vi "Thermal Cam Standalone.vi"() -> ()   [LabVIEW 2025]
uses:
  CTI/Identity.ctl
  Colormaps/LV Colormap Names.ctl
  CTI/GPIO Pull.ctl
  45a22dfa-6e5d-42d3-9540-e99b2dd074d1.vi
  1e6ec9c9-fb05-4fd0-b05f-9caec19ae962.vi
  8524c294-126d-4a78-a4f4-5e8209367d85.vi
  7e432e81-cfec-40ee-91ac-c41f46aea1a5.vi
  81a0c2b0-cfce-4e0a-bc55-b9605872672a.vi
  <vilib>/gmath/interp.llb/Interpolate 2D (2d X,Y).vi
  CTI/Session/Session.lvclass
  <vilib>/gmath/NI_Gmath.lvlib
  <vilib>/ptbypt/NI_PtbyPt.lvlib
  CTI/VisaComms/VisaComms.lvclass
  CTI/CTI.lvlib
panel:
  in  "Interpolate":bool=TRUE
  in  "Max hold":bool
  in  "Temperature\nCompression":dbl=3.0
  in  "Auto Z Scale":bool=TRUE
  out "Average Max":dbl=82.15301832388433 format="%.1f"
  out "Current Max":dbl=82.15301832388433 format="%.1f"
  in  "Exponentional\nAveraging Alpha":dbl=0.4 min=0.0 max=1.0 step=0.05 format="%#_13g"
  in  "Temperature\nDispalyRange":dbl=12.0
  in  "Smoothing \nMethod":i32(ring)=3 items=["nearest", "bilinear", "bicubic", "bicubic spline"]
  in  "Colormap Name":T1=enum."turbo"
  in  "Stop":bool
  out "Unprocessed Pixels":dbl[][](graph)
  out "Interpolated Frame":dbl[][](graph)
  out "Processing Performance":dbl(graph)=0.0211100999986229
  out "Identity":T2
  out "On-board\nTempSensor":dbl
  out "Frame Count":i32
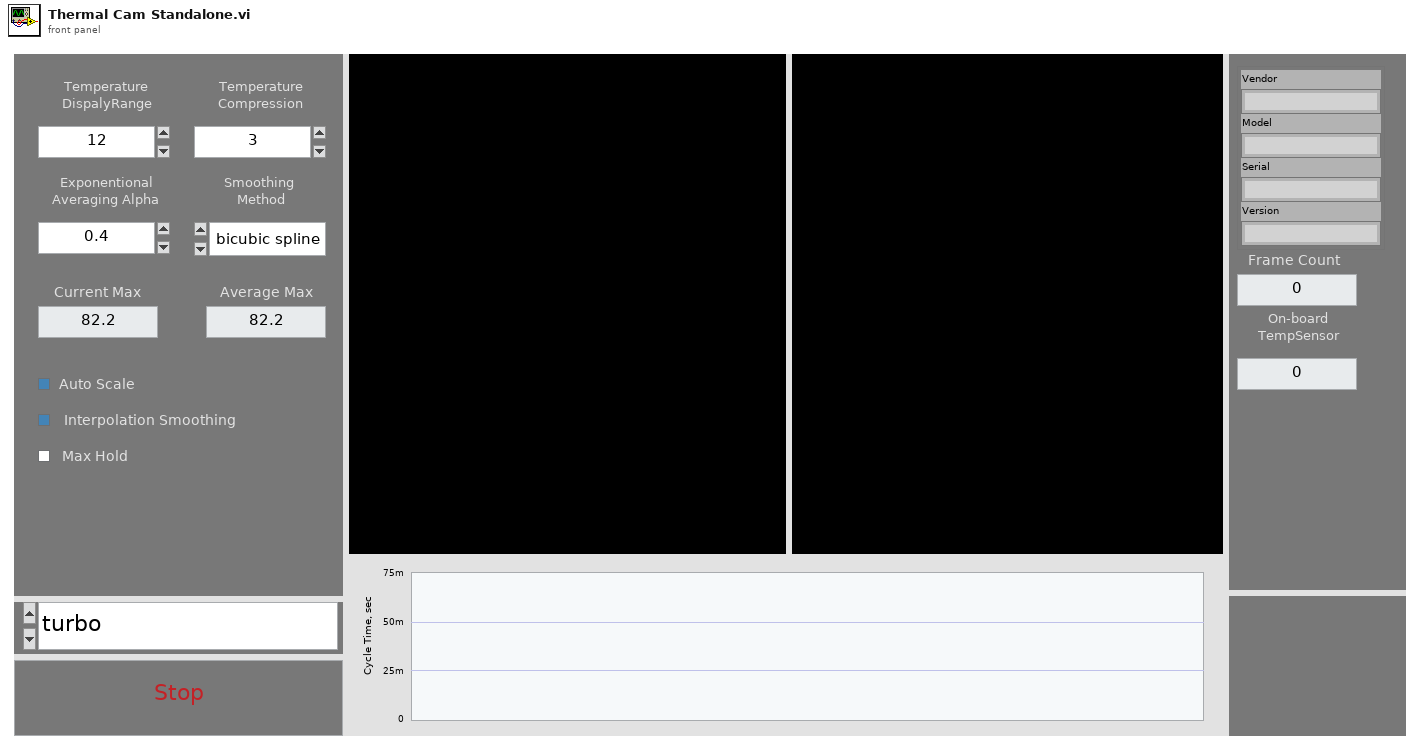
[diagram p1: front panel]
types:
  T1 = typedef "LV Colormap Names.ctl" = enum16{"Accent", "Accent_r", "Blues", "Blues_r", "BrBG", "BrBG_r", "BuGn", "BuGn_r", "BuPu", "BuPu_r", "CMRmap", "CMRmap_r", "Dark2", "Dark2_r", "GnBu", "GnBu_r", "Grays", "Grays_r", "Greens", "Greens_r", "Greys", "Greys_r", "OrRd", "OrRd_r", "Oranges", "Oranges_r", "PRGn", "PRGn_r", "Paired", "Paired_r", "Pastel1", "Pastel1_r", "Pastel2", "Pastel2_r", "PiYG", "PiYG_r", "PuBu", "PuBuGn", "PuBuGn_r", "PuBu_r", "PuOr", "PuOr_r", "PuRd", "PuRd_r", "Purples", "Purples_r", "RdBu", "RdBu_r", "RdGy", "RdGy_r", "RdPu", "RdPu_r", "RdYlBu", "RdYlBu_r", "RdYlGn", "RdYlGn_r", "Reds", "Reds_r", "Set1", "Set1_r", "Set2", "Set2_r", "Set3", "Set3_r", "Spectral", "Spectral_r", "Wistia", "Wistia_r", "YlGn", "YlGnBu", "YlGnBu_r", "YlGn_r", "YlOrBr", "YlOrBr_r", "YlOrRd", "YlOrRd_r", "afmhot", "afmhot_r", "autumn", "autumn_r", "berlin", "berlin_r", "binary", "binary_r", "bone", "bone_r", "brg", "brg_r", "bwr", "bwr_r", "cividis", "cividis_r", "cool", "cool_r", "coolwarm", "coolwarm_r", "copper", "copper_r", "cubehelix", "cubehelix_r", "flag", "flag_r", "gist_earth", "gist_earth_r", "gist_gray", "gist_gray_r", "gist_grey", "gist_grey_r", "gist_heat", "gist_heat_r", "gist_ncar", "gist_ncar_r", "gist_rainbow", "gist_rainbow_r", "gist_stern", "gist_stern_r", "gist_yarg", "gist_yarg_r", "gist_yerg", "gist_yerg_r", "gnuplot", "gnuplot2", "gnuplot2_r", "gnuplot_r", "gray", "gray_r", "grey", "grey_r", "hot", "hot_r", "hsv", "hsv_r", "inferno", "inferno_r", "jet", "jet_r", "magma", "magma_r", "managua", "managua_r", "nipy_spectral", "nipy_spectral_r", "ocean", "ocean_r", "pink", "pink_r", "plasma", "plasma_r", "prism", "prism_r", "rainbow", "rainbow_r", "seismic", "seismic_r", "spring", "spring_r", "summer", "summer_r", "tab10", "tab10_r", "tab20", "tab20_r", "tab20b", "tab20b_r", "tab20c", "tab20c_r", "terrain", "terrain_r", "turbo", "turbo_r", "twilight", "twilight_r", "twilight_shifted", "twilight_shifted_r", "vanimo", "vanimo_r", "viridis", "viridis_r", "winter", "winter_r"}
  T2 = typedef "CTI.lvlib/Identity.ctl" = cluster{"Vendor":string, "Model":string, "Serial":string, "Version":string}
  T3 = typedef "CTI.lvlib/GPIO Pull.ctl" = enum16{"None", "Up", "Down", "Both"}
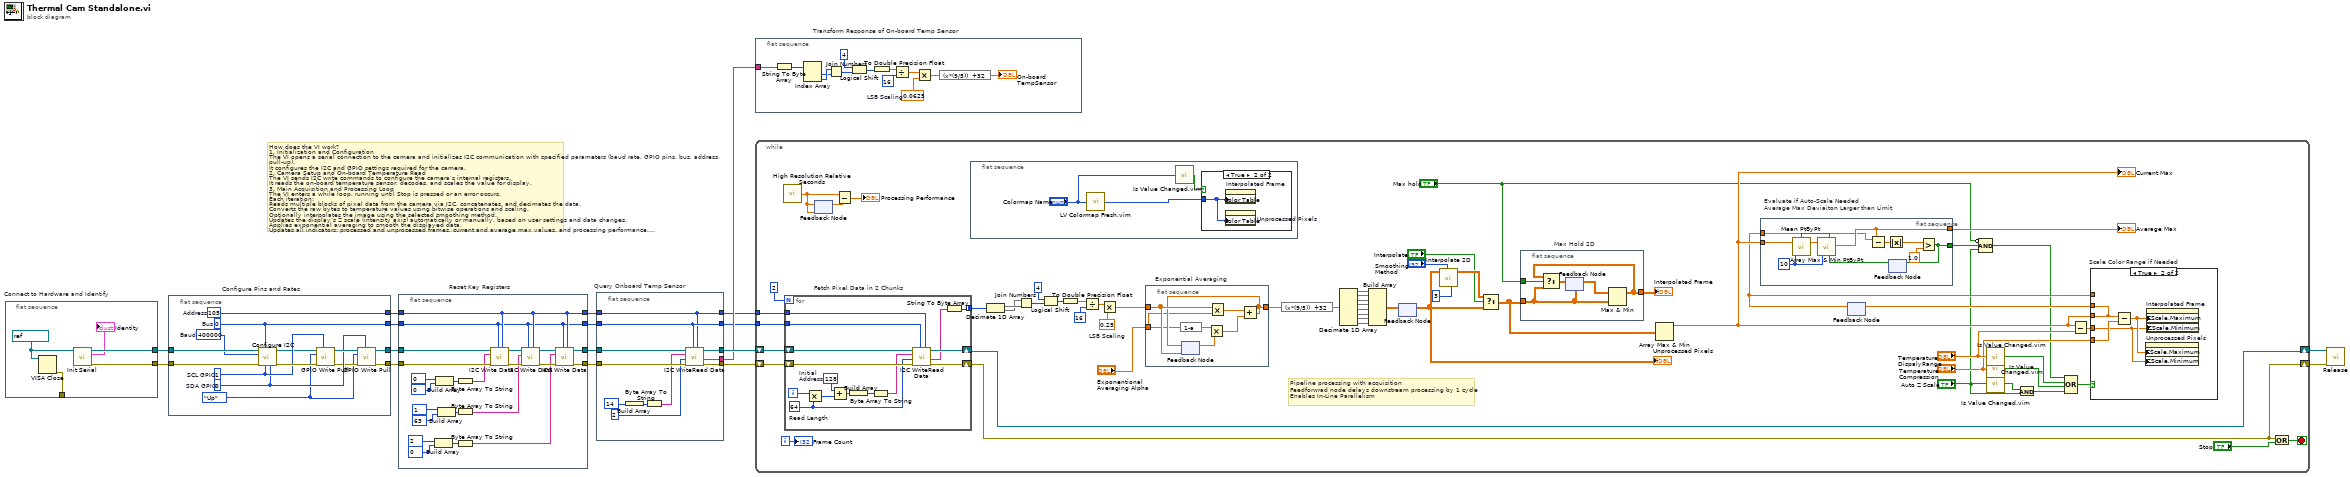
[diagram p0: block diagram]
diagram:
  # "How does the VI work?\n1. Initialization and Configuration\nThe VI opens a serial connection to the camera and initializes I2C communication with specified parameters (baud rate, GPIO pins, bus, address, pull-up).\nIt configures the I2C and GPIO settings required for the camera.\n2. Camera Setup and On-board Temperature Read\nThe VI sends I2C write commands to configure the camera’s internal registers.\nIt reads the on-board temperature sensor, decodes, and scales the value for display.\n3. Main Acquisition and Processing Loop\nThe VI enters a while loop, running until Stop is pressed or an error occurs.\nEach iteration:\nReads multiple blocks of pixel data from the camera via I2C, concatenates, and decimates the data.\nConverts the raw bytes to temperature values using bitwise operations and scaling.\nOptionally interpolates the image using the selected smoothing method.\nUpdates the display’s Z scale (intensity axis) automatically or manually, based on user settings and data changes.\nApplies exponential averaging to smooth the displayed data.\nUpdates all indicators: processed and unprocessed frames, current and average max values, and processing performance.\n4. Visualization\nThe VI updates the color map of the intensity graph if the user changes the colormap.\nIt provides options for interpolation, auto-scaling, and maximum hold to enhance visualization.\n5. Cleanup\nAfter the loop, the VI releases the camera session and cleans up resources."
  n1 = flat-sequence "Connect to Hardware and Identify" {
    tunnel: [w22] -> w17
    tunnel: [w21] -> w16
    tunnel: [w18] -> _
    frame #0 {
      w19 = refnum<visa-resource-name> "COM9" ("VISA resource name in")
      n2 = VISA Close(VISA resource name=w19) -> (error out=w18:errorcluster)  [unwired: 1 in]
      n3 = call "Init Serial.vi"("VISA resource name in"=w19) -> ("error out"=w21:errorcluster, "Identity"=→"Identity":T2, "Session"=w22:refnum<class "Session.lvclass">)  [unwired: 8 in]
    }
  }
  n4 = flat-sequence "Configure Pins and Rates" {
    tunnel: w17 -> [w36]
    tunnel: w16 -> [w35]
    tunnel: [w28] -> w15
    tunnel: [w27] -> w14
    tunnel: [w26] -> w9
    tunnel: [w25] -> w8
    frame #0 {
      w23 = GPIO_Pull."Up" ("GPIO Pull")
      w25 = u8 105  # Address
      w26 = u8 0  # Bus
      w31 = 1  # SCL GPIO
      w30 = 0  # SDA GPIO
      w34 = u32 400000  # Baud
      n5 = call "Configure I2C.vi"("SDA GPIO"=w30, "SCL GPIO"=w31, "I2C #"=w26, "error in (no error)"=w35, "Baud"=w34, "Session in"=w36) -> ("error out"=w33:errorcluster, "Session out"=w24:refnum<class "Session.lvclass">)  [unwired: 4 in]
      n6 = call "GPIO Write Pull.vi"("GPIO #"=w31, "error in (no error)"=w33, "GPIO Pull"=w23, "Session in"=w24) -> ("error out"=w29:errorcluster, "Session out"=w32:refnum<class "Session.lvclass">)  [unwired: 6 in]
      n7 = call "GPIO Write Pull.vi"("GPIO #"=w30, "error in (no error)"=w29, "GPIO Pull"=w23, "Session in"=w32) -> ("error out"=w28:errorcluster, "Session out"=w27:refnum<class "Session.lvclass">)  [unwired: 6 in]
    }
  }
  n8 = flat-sequence "Reset Key Registers" {
    tunnel: w15 -> [w58]
    tunnel: w14 -> [w57]
    tunnel: [w45] -> w13
    tunnel: [w39] -> w11
    tunnel: w9 -> [w37]
    tunnel: w8 -> [w38]
    tunnel: [w38] -> w6
    tunnel: [w37] -> w5
    frame #0 {
      n9 = Build Array(u8 2 ("Address"), u8 0 ("Address")) -> (w41:u8[])
      n10 = Build Array(u8 0 ("Address"), u8 0 ("Address")) -> (w53:u8[])
      n11 = Build Array(u8 1 ("Address"), u8 63 ("Address")) -> (w49:u8[])
      n12 = Byte Array To String(unsigned byte array=w53) -> (string=w56:string)
      n13 = Byte Array To String(unsigned byte array=w49) -> (string=w46:string)
      n14 = Byte Array To String(unsigned byte array=w41) -> (string=w40:string)
      n15 = call "I2C Write Data.vi"("Address"=w38, "I2C #"=w37, "error in (no error)"=w58, "Data"=w56, "Session in"=w57) -> ("error out"=w52:errorcluster, "Session out"=w50:refnum<class "Session.lvclass">)  [unwired: 5 in]
      n16 = call "I2C Write Data.vi"("Address"=w38, "I2C #"=w37, "error in (no error)"=w52, "Data"=w46, "Session in"=w50) -> ("error out"=w51:errorcluster, "Session out"=w44:refnum<class "Session.lvclass">)  [unwired: 5 in]
      n17 = call "I2C Write Data.vi"("Address"=w38, "I2C #"=w37, "error in (no error)"=w51, "Data"=w40, "Session in"=w44) -> ("error out"=w45:errorcluster, "Session out"=w39:refnum<class "Session.lvclass">)  [unwired: 5 in]
    }
  }
  n18 = flat-sequence "Query Onboard Temp Sensor" {
    tunnel: w13 -> [w69]
    tunnel: [w68] -> w12
    tunnel: w11 -> [w67]
    tunnel: [w66] -> w10
    tunnel: w5 -> [w60]
    tunnel: w6 -> [w59]
    tunnel: [w62] -> w7
    tunnel: [w60] -> w4
    tunnel: [w59] -> w3
    frame #0 {
      n19 = Build Array(u8 14 ("Address")) -> (w64:u8[])
      n20 = Byte Array To String(unsigned byte array=w64) -> (string=w63:string)
      n21 = call "I2C WriteRead Data.vi"("Address"=w59, "I2C #"=w60, "error in (no error)"=w69, "Len"=u8 2 ("Read Len"), "Write Data"=w63, "Session in"=w67) -> ("error out"=w68:errorcluster, "Read Data"=w62:string, "Session out"=w66:refnum<class "Session.lvclass">)  [unwired: 3 in]
    }
  }
  n22 = while {
    tunnel: w4 -> [w115]
    tunnel: w3 -> [w114]
    shift-right: [w76] -> w1
    shift-left: w12 -> [w117]
    shift-right: [w79] -> w2
    shift-left: w10 -> [w116]
    i -> [w113]
    stop <- w112 stop-if-true
    w100 = 0.25  # LSB Scaling
    # "Pipeline processing with acquisition\nFeedforwrad node delays downstream processing by 1 cycle\nEnables In-Line Parallelism"
    n23 = call <vilib>:"High Resolution Relative Seconds.vi"() -> ("relative seconds"=w104:dbl)
    n24 = for "Fetch Pixel Data in 2 Chunks" {
      N: 2 -> [_]
      shift-right: [w165] -> w76
      shift-left: w117 -> [w166]
      shift-right: [w164] -> w79
      shift-left: w116 -> [w167]
      tunnel: w115 -> [w163]
      tunnel: w114 -> [w162]
      tunnel: [w168] -> w128 mode=concatenating
      i -> [w157]
      w158 = u8 64  # Read Length
      w159 = u8 128  # Initial Address
      n25 = Multiply(x=w157, y=w158) -> (x*y=w155:i32)
      n26 = Add(x=w159, y=w155) -> (x+y=w156:i32)
      n27 = Build Array(w156) -> (w169:i32[])
      n28 = Byte Array To String(unsigned byte array=w169) -> (string=w161:string)
      n29 = call "I2C WriteRead Data.vi"("Address"=w162, "I2C #"=w163, "error in (no error)"=w166, "Len"=w158, "Write Data"=w161, "Session in"=w167) -> ("error out"=w165:errorcluster, "Read Data"=w160:string, "Session out"=w164:refnum<class "Session.lvclass">)  [unwired: 3 in]
      n30 = String To Byte Array(string=w160) -> (unsigned byte array=w168:u8[])
    }
    n31 = feedback-in #1(w104) -> ()
    n32 = feedback #1(w104) -> (w103:dbl)
    n33 = Subtract(x=w104, y=w103) -> (x-y=→"Processing Performance":dbl)
    n34 = flat-sequence {
      frame #0 {
        n35 = call "LV Colormap Fresh.vim"("Colormap Name"="Colormap Name") -> ("Colormap"=w145:u32[])  [unwired: 14 in]
        n36 = call "Is Value Changed.vim"("value"="Colormap Name") -> ("changed or first call?"=w146:bool)
        n37 = case shown="True" w146 {
          tunnel: w145 -> [_ w147]
          frame False {
          }
          frame True {
            n38 = property on="Interpolated Frame" class="IntGraph (strict)"("Color Table"=w147) -> ()  [unwired: 2 in, 2 out]
            n39 = property on="Unprocessed Pixels" class="IntGraph (strict)"("Color Table"=w147) -> ()  [unwired: 2 in, 2 out]
          }
        }
      }
    }
    n40 = Decimate 1D Array(w128) -> (w127:u8[], w126:u8[])
    n41 = Join Numbers(hi=w126, lo=w127) -> ((hi.lo)=w107:u16[])
    n42 = Logical Shift(y=i16 4, x=w107) -> (x << y=w110:u16[])
    n43 = To Double Precision Float(number=w110) -> (double precision float=w109:dbl[])
    n44 = Divide(x=w109, y=i16 16) -> (x/y=w106:dbl[])
    n45 = Multiply(x=w106, y=w100) -> (x*y=w98:dbl[])
    n46 = flat-sequence "Exponential Averaging" {
      tunnel: w98 -> [w150]
      tunnel: [w149] -> w97
      tunnel: "Exponentional\nAveraging Alpha" -> [w148]
      frame #0 {
        n47 = expression code="1-a"(w148) -> (w153:dbl)
        n48 = feedback #2(w150) -> (w151:dbl[])
        n49 = Multiply(x=w153, y=w151) -> (x*y=w152:dbl[])
        n50 = Multiply(x=w150, y=w148) -> (x*y=w154:dbl[])
        n51 = Add(x=w154, y=w152) -> (x+y=w149:dbl[])
        n52 = feedback-in #2(w149) -> ()
      }
    }
    n53 = expression code="(x*(9/5))  +32"(w97) -> (w105:dbl[])
    n54 = Decimate 1D Array(w105) -> (w118:dbl[], w119:dbl[], w120:dbl[], w121:dbl[], w122:dbl[], w123:dbl[], w124:dbl[], w125:dbl[])
    n55 = Build Array(w118, w119, w120, w121, w122, w123, w124, w125) -> (w80:dbl[][])
    n56 = feedback-in #3(w80) -> ()
    n57 = feedback #3() -> (w75:dbl[][])  [unwired: 1 in]
    "Unprocessed Pixels" <- w75
    n58 = call-poly <vilib>:"Interpolate 2D.vi"("ntimes"=3, "method"="Smoothing \nMethod", "Z"=w75) -> ("zi"=w90:dbl[][])  [unwired: 5 in, 3 out]
    n59 = Select(t=w90, s="Interpolate", f=w75) -> (s? t:f=w89:dbl[][])
    n60 = flat-sequence "Max Hold 2D" {
      tunnel: [w132] -> w91
      tunnel: w89 -> [w130]
      tunnel: "Max hold" -> [w129]
      frame #0 {
        n61 = feedback #4(w130) -> (w133:dbl[][])
        n62 = Max & Min(x=w133, y=w130) -> (max(x,y)=w132:dbl[][])  [unwired: 1 out]
        n63 = Select(t=w132, s=w129, f=w130) -> (s? t:f=w131:dbl[][])
        n64 = feedback-in #4(w131) -> ()
      }
    }
    n65 = Array Max & Min(array=w89) -> (max value=w92:dbl)  [unwired: 3 out]
    "Current Max" <- w92
    n66 = flat-sequence "Evaluate if Auto-Scale Needed\nAverage Max Deviaiton Larger than Limit" {
      tunnel: [w137] -> w94
      tunnel: w92 -> [w136]
      tunnel: w77 -> [w135]
      tunnel: [w134] -> w83
      frame #0 {
        w139 = 10 ("sample length")
        n67 = feedback #5() -> (w138:bool)  [unwired: 1 in]
        n68 = call <vilib>:"Mean PtByPt.vi"("x"=w136, "sample length"=w139, "initialize"=w138) -> ("mean"=w140:dbl)  [unwired: 1 in, 1 out]
        n69 = call <vilib>:"Array Max & Min PtByPt.vi"("input data point"=w140, "sample length"=w139, "initialize"=w138) -> ("max value"=w137:dbl)  [unwired: 4 out]
        n70 = Subtract(x=w135, y=w137) -> (x-y=w143:dbl)
        n71 = Absolute Value(x=w143) -> (abs(x)=w142:dbl)
        n72 = Greater?(x=w142, y=1.0) -> (0:w134:bool)
        n73 = feedback-in #5(w134) -> ()
      }
    }
    n74 = feedback #6() -> (w77:dbl)  [unwired: 1 in]
    n75 = Compound Arithmetic op=AND(invert "Max hold", w83, "Auto Z Scale") -> (w73:bool)
    n76 = call "Is Value Changed.vim"("value"="Temperature\nDispalyRange") -> ("changed or first call?"=w95:bool)
    n77 = call "Is Value Changed.vim"("value"="Temperature\nCompression") -> ("changed or first call?"=w86:bool)
    n78 = call "Is Value Changed.vim"("value"="Auto Z Scale") -> ("changed or first call?"=w85:bool)
    n79 = And(x=w85, y="Auto Z Scale") -> (x .and. y?=w71:bool)
    n80 = Compound Arithmetic op=OR(w73, w95, w86, w71) -> (w72:bool)
    n81 = Subtract(x=w92, y="Temperature\nDispalyRange") -> (x-y=w99:dbl)
    n82 = case "Scale Color Range if Needed" shown="True" w72 {
      tunnel: w99 -> [_ w171]
      tunnel: w92 -> [_ w174]
      tunnel: [w170 w174] -> w93
      tunnel: w77 -> [w170 _]
      tunnel: "Temperature\nCompression" -> [_ w173]
      frame False {
      }
      frame True {
        n83 = Subtract(x=w174, y=w173) -> (x-y=w172:dbl)
        n84 = property on="Unprocessed Pixels" class="IntGraph (strict)"("ZScale.Maximum"=w172, "ZScale.Minimum"=w171) -> ()  [unwired: 2 in, 2 out]
        n85 = property on="Interpolated Frame" class="IntGraph (strict)"("ZScale.Maximum"=w172, "ZScale.Minimum"=w171) -> ()  [unwired: 2 in, 2 out]
      }
    }
    n86 = feedback-in #6(w93) -> ()
    n87 = Or(x=w76, y="Stop") -> (x .or. y?=w112:bool)
    "Interpolated Frame" <- w91
    "Frame Count" <- w113
    "Average Max" <- w94
  }
  n88 = flat-sequence "Transform Response of On-board Temp Sensor" {
    tunnel: w7 -> [w187]
    frame #0 {
      w175 = 0.0625  # LSB Scaling
      n89 = String To Byte Array(string=w187) -> (unsigned byte array=w186:u8[])
      n90 = Index Array(array=w186) -> (element #1=w184:u8, element #2=w185:u8)  [unwired: 2 in]
      n91 = Join Numbers(hi=w185, lo=w184) -> ((hi.lo)=w177:u16)
      n92 = Logical Shift(y=i16 4, x=w177) -> (x << y=w180:u16)
      n93 = To Double Precision Float(number=w180) -> (double precision float=w181:dbl)
      n94 = Divide(x=w181, y=i16 16) -> (x/y=w183:dbl)
      n95 = Multiply(x=w183, y=w175) -> (x*y=w176:dbl)
      n96 = expression code="(x*(9/5))  +32"(w176) -> (→"On-board\nTempSensor":dbl)
    }
  }
  n97 = call-dynamic "Release.vi"("error in (no error)"=w1, "Session in"=w2) -> ()  [unwired: 9 in, 1 out]
